vi "Periodic Tasks.vi"(8 "error in":errorcluster) -> ()   [LabVIEW 2014]
doc: "This VI runs in parallel to other tasks. It can contain as many user-defined periodic loops as you need. These can carry out PID or other sorts of timed response."
uses:
  TypeDefs/SRE Enum.ctl
  <vilib>/Rock Robotics/Network Tables/SD Write Number.vi
  Robot Global Data.vi
  Get Ctrl/Get ctrl Secondary axis.vi
  Get Ctrl/Get ctrl Secondary Button.vi
panel:
  in  "Lift to Running":bool
  out "Enum":enum16{"In", "Out", "Done"}(ring)
  in  "Max Change":dbl=0.1
  in  "Stall Speed":dbl=0.05
  out "Angle":dbl
  out "Arm Pot":dbl
  out "Lift Pot":dbl
  out "current (A)":dbl
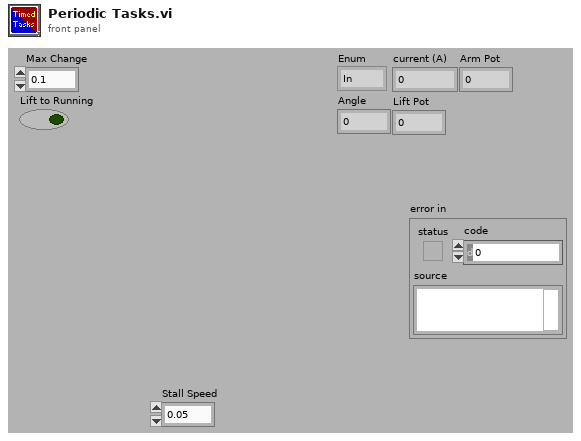
[diagram p1: front panel]
types:
  T1 = enum16{"High", "Middle", "Low", "Really Low", "Stopped"}
  T2 = typedef "SRE Enum.ctl" = enum16{"Start", "Run", "End"}
  T3 = cluster{"proportional gain (Kc)":dbl, "derivative time (Td, min)":dbl}
  T4 = enum16{"manual Control of arm", "manual Control of Elevator", "Output Control"}[]
  T5 = cluster{"Speed":dbl, "Direction":dbl, "Rotation":dbl}
  T6 = enum16{"Auto Stack", "Claw up", "Enable Manuel Elevator", "EM Claw", "Open Claw"}[]
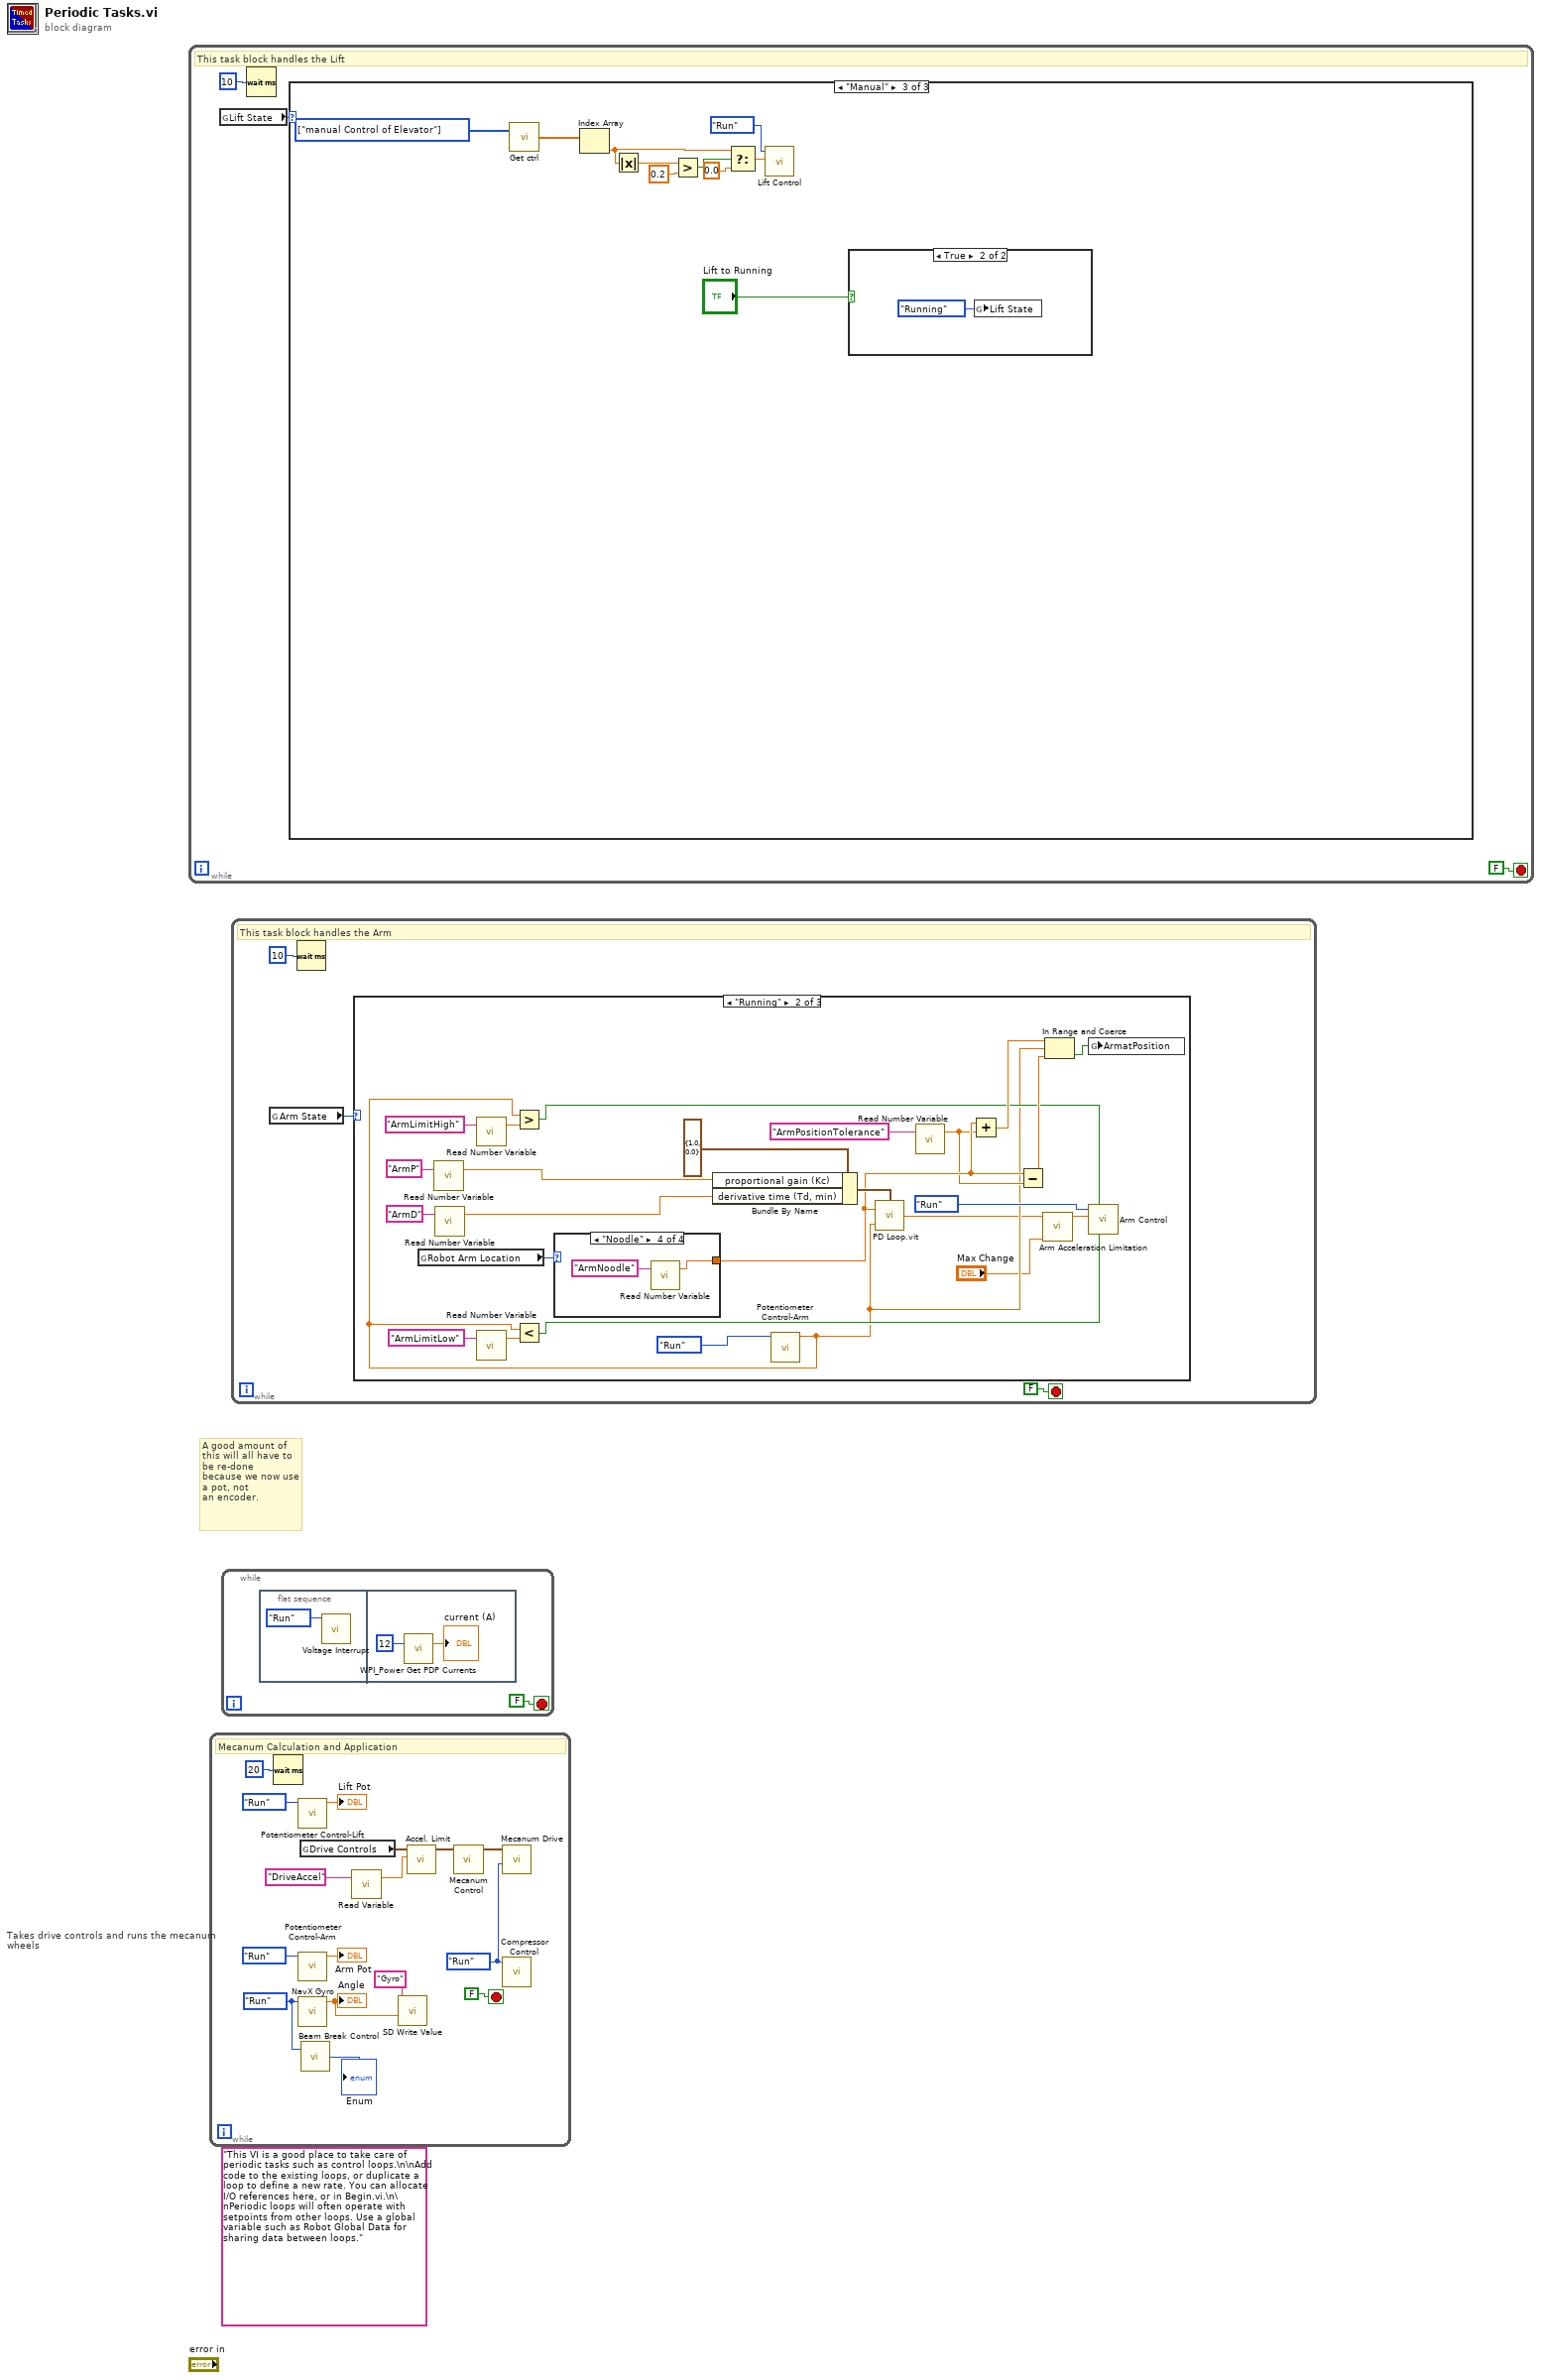
[diagram p0: block diagram]
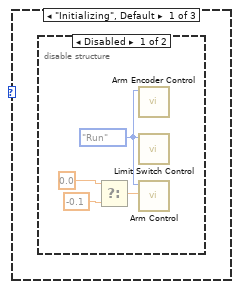
[diagram p2: hidden frame]
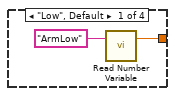
[diagram p4: hidden frame]
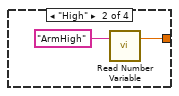
[diagram p5: hidden frame]
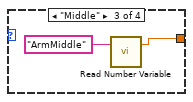
[diagram p6: hidden frame]
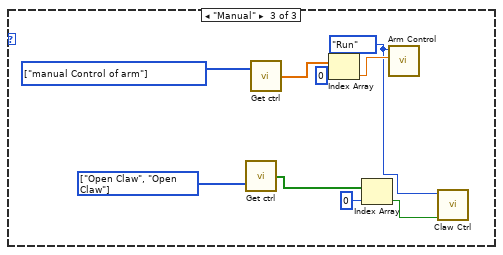
[diagram p7: hidden frame]
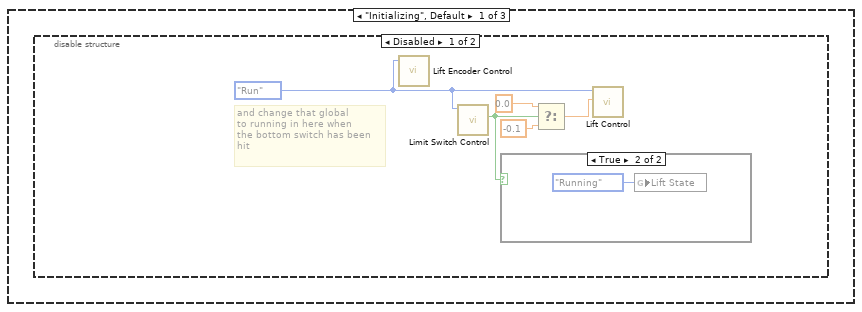
[diagram p8: hidden frame]
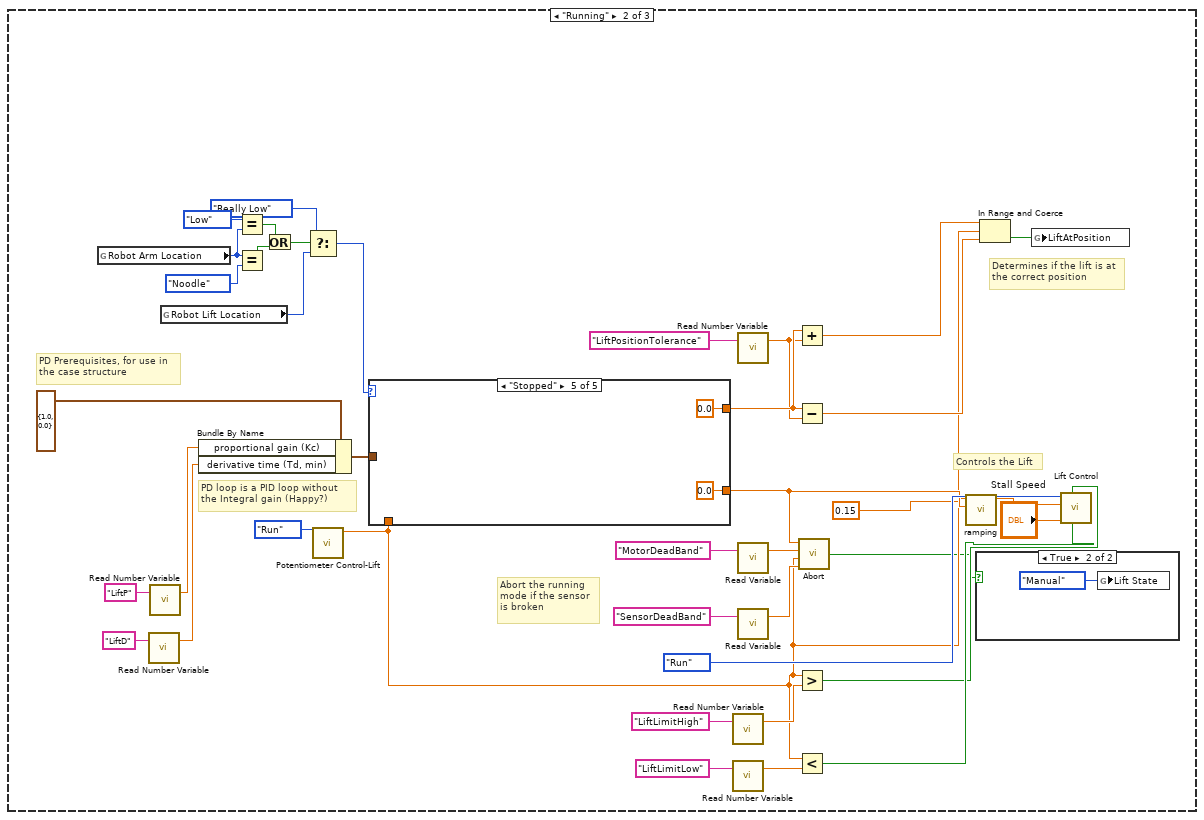
[diagram p11: hidden frame]
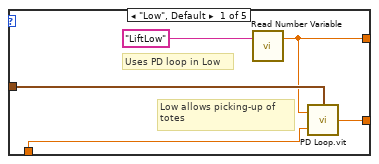
[diagram p13: hidden frame]
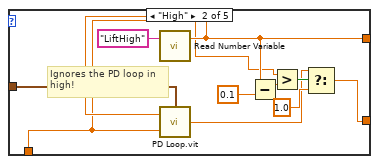
[diagram p14: hidden frame]
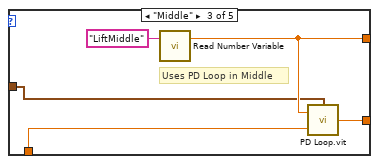
[diagram p15: hidden frame]
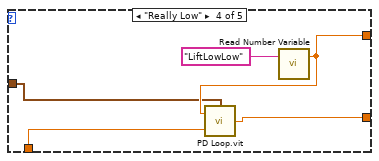
[diagram p16: hidden frame]
diagram:
  (unwired) "This VI is a good place to take care of periodic tasks such as control loops.\n\nAdd code to the existing loops, or duplicate a loop to define a new rate. You can allocate I/O references here, or in Begin.vi.\n\nPeriodic loops will often operate with setpoints from other loops. Use a global variable such as Robot Global Data for sharing data between loops."
  # "A good amount of this will all have to be re-done\nbecause we now use a pot, not\nan encoder."
  n1 = while {
    stop <- FALSE stop-if-true
    # "This task block handles the Lift"
    n2 = global read "Robot Global Data.vi" "Lift State"() -> (w1:enum16{"Initializing", "Running", "Manual"})
    n3 = Wait (ms)(milliseconds to wait=u32 10) -> ()  [unwired: 1 out]
    n4 = case shown="\"Manual\"" w1 {
      frame "Initializing", Default {
        n5 = disable-structure shown="Disabled" {
          frame Disabled {
            w6 = SRE_Enum."Run" ("Enum")
            # "and change that global\nto running in here when\nthe bottom switch has been\nhit"
            n6 = call "Lift Encoder Control.vi"("Enum"=w6) -> ()  [unwired: 6 in, 2 out]
            n7 = call "Limit Switch Control.vi"("Run Mode"=w6) -> ("Lift Bottom"=w4:bool)  [unwired: 7 in, 3 out]
            n8 = case shown="True" w4 {
              frame False {
              }
              frame True {
                n9 = global write "Robot Global Data.vi" "Lift State"(enum16{"Initializing", "Running", "Manual"}."Running" ("Lift State")) -> ()
              }
            }
            n10 = Select(t=0.0, s=w4, f=-0.1) -> (s? t:f=w5:dbl)
            n11 = call "Lift Control.vi"("Motor"=w5, "Enum"=w6) -> ()  [unwired: 9 in, 1 out]
          }
          frame Enabled {
          }
        }
      }
      frame "Running" {
        # "Abort the running\nmode if the sensor\nis broken"
        # "Controls the Lift"
        # "PD loop is a PID loop without\nthe Integral gain (Happy?)"
        # "Determines if the lift is at\nthe correct position"
        # "PD Prerequisites, for use in\nthe case structure"
        n12 = global read "Robot Global Data.vi" "Robot Arm Location"() -> (w20:enum16{"High", "Middle", "Low", "Noodle"})
        n13 = call "Read Number Variable.vi"("Name"="LiftD") -> ("number"=w21:dbl)  [unwired: 1 in, 1 out]
        n14 = call "Read Number Variable.vi"("Name"="LiftP") -> ("number"=w22:dbl)  [unwired: 1 in, 1 out]
        n15 = global read "Robot Global Data.vi" "Robot Lift Location"() -> (w14:T1)
        n16 = Bundle By Name(cluster=T3 {"proportional gain (Kc)"=1.0, "derivative time (Td, min)"=0.0} ("PID gains"), "proportional gain (Kc)"=w22, "derivative time (Td, min)"=w21) -> (w28:T3)
        n17 = Equal?(x=enum16{"High", "Middle", "Low", "Noodle"}."Low", y=w20) -> (x = y?=w16:bool)
        n18 = Equal?(x=w20, y=enum16{"High", "Middle", "Low", "Noodle"}."Noodle") -> (x = y?=w17:bool)
        n19 = Or(x=w16, y=w17) -> (x .or. y?=w15:bool)
        n20 = Select(t=T1."Really Low", s=w15, f=w14) -> (s? t:f=w12:T1)
        n21 = call "Potentiometer Control-Lift.vi"("Enum"=SRE_Enum."Run") -> ("Normalized Value"=w11:dbl)  [unwired: 10 in]
        n22 = case shown="\"Stopped\"" w12 {
          tunnel: [w51 w59 w68 w72 0.0 ("number")] -> w44
          tunnel: w28 -> [w52 w60 w67 w71 _]
          tunnel: [w53 w61 w66 w70 0.0 ("Out Power")] -> w27
          tunnel: w11 -> [w50 w58 w65 w73 _]
          frame "Low", Default {
            # "Low allows picking-up of\ntotes"
            # "Uses PD loop in Low"
            n23 = call "Read Number Variable.vi"("Name"="LiftLow") -> ("number"=w51:dbl)  [unwired: 1 in, 1 out]
            n24 = call "PD Loop.vit"("PD Gains"=w52, "Current"=w50, "Set"=w51) -> ("Out Power"=w53:dbl)
          }
          frame "High" {
            # "Ignores the PD loop in\nhigh!"
            n25 = call "Read Number Variable.vi"("Name"="LiftHigh") -> ("number"=w59:dbl)  [unwired: 1 in, 1 out]
            n26 = call "PD Loop.vit"("PD Gains"=w60, "Current"=w58, "Set"=w59) -> ("Out Power"=w57:dbl)
            n27 = Subtract(x=w59, y=0.1) -> (x-y=w56:dbl)
            n28 = Greater?(x=w58, y=w56) -> (0:w63:bool)
            n29 = Select(t=w57, s=w63, f=1.0) -> (s? t:f=w61:dbl)
          }
          frame "Middle" {
            # "Uses PD Loop in Middle"
            n30 = call "Read Number Variable.vi"("Name"="LiftMiddle") -> ("number"=w68:dbl)  [unwired: 1 in, 1 out]
            n31 = call "PD Loop.vit"("PD Gains"=w67, "Current"=w65, "Set"=w68) -> ("Out Power"=w66:dbl)
          }
          frame "Really Low" {
            n32 = call "Read Number Variable.vi"("Name"="LiftLowLow") -> ("number"=w72:dbl)  [unwired: 1 in, 1 out]
            n33 = call "PD Loop.vit"("PD Gains"=w71, "Current"=w73, "Set"=w72) -> ("Out Power"=w70:dbl)
          }
          frame "Stopped" {
          }
        }
        n34 = call "Read Number Variable.vi"("Name"="LiftLimitHigh") -> ("number"=w46:dbl)  [unwired: 1 in, 1 out]
        n35 = call "Read Number Variable.vi"("Name"="LiftLimitLow") -> ("number"=w45:dbl)  [unwired: 1 in, 1 out]
        n36 = call "Read Number Variable.vi"("Name"="LiftPositionTolerance") -> ("number"=w42:dbl)  [unwired: 1 in, 1 out]
        n37 = call-poly "Read Variable.vi"("Name"="MotorDeadBand") -> ("number"=w38:dbl)  [unwired: 1 in, 1 out]
        n38 = call-poly "Read Variable.vi"("Name"="SensorDeadBand") -> ("number"=w39:dbl)  [unwired: 1 in, 1 out]
        n39 = Add(x=w44, y=w42) -> (x+y=w36:dbl)
        n40 = Subtract(x=w44, y=w42) -> (x-y=w35:dbl)
        n41 = Greater?(x=w11, y=w46) -> (0:w32:bool)
        n42 = Less?(x=w11, y=w45) -> (x < y?=w33:bool)
        n43 = call "Abort.vi"("Sensor Deadband"=w39, "Sensor"=w11, "Motor Deadband"=w38, "Motor"=w27) -> ("Abort"=w10:bool)
        n44 = call "ramping.vi"("Speed"=w27, "Max Change"=0.15) -> ("New Speed"=w26:dbl)  [unwired: 9 in]
        n45 = case shown="True" w10 {
          frame False {
          }
          frame True {
            n46 = global write "Robot Global Data.vi" "Lift State"(enum16{"Initializing", "Running", "Manual"}."Manual" ("Lift State")) -> ()
          }
        }
        n47 = In Range and Coerce(upper limit=w36, x=w11, lower limit=w35) -> (In Range?=w34:bool)  [unwired: 1 out]
        n48 = global write "Robot Global Data.vi" "LiftAtPosition"(w34) -> ()
        n49 = call "Lift Control.vi"("bottom"=w33, "top"=w32, "Stall Speed"="Stall Speed", "Motor"=w26, "Enum"=SRE_Enum."Run") -> ()  [unwired: 6 in, 1 out]
      }
      frame "Manual" {
        w78 = T4 [enum."manual Control of Elevator"] items=["manual Control of arm", "manual Control of Elevator", "Output Control"] ("TypeDef")
        n50 = call-poly "Get ctrl.vi"("TypeDef"=w78) -> ("Array"=w85:dbl[])  [unwired: 2 in]
        n51 = Index Array(array=w85) -> (element=w81:dbl)  [unwired: 1 in]
        n52 = Absolute Value(x=w81) -> (abs(x)=w84:dbl)
        n53 = Greater?(x=w84, y=0.2) -> (0:w82:bool)
        n54 = Select(t=w81, s=w82, f=0.0) -> (s? t:f=w79:dbl)
        n55 = call "Lift Control.vi"("Motor"=w79, "Enum"=SRE_Enum."Run") -> ()  [unwired: 9 in, 1 out]
        n56 = case shown="True" "Lift to Running" {
          frame False {
          }
          frame True {
            n57 = global write "Robot Global Data.vi" "Lift State"(enum16{"Initializing", "Running", "Manual"}."Running" ("Lift State")) -> ()
          }
        }
      }
    }
  }
  n58 = while "Takes drive controls and runs the mecanum wheels" {
    stop <- FALSE stop-if-true
    w89 = SRE_Enum."Run" ("Enum")
    w96 = SRE_Enum."Run" ("Enum")
    # "Mecanum Calculation and Application"
    n59 = Wait (ms)(milliseconds to wait=u32 20) -> ()  [unwired: 1 out]
    n60 = call "Potentiometer Control-Lift.vi"("Enum"=SRE_Enum."Run") -> ("Normalized Value"=→"Lift Pot":dbl)  [unwired: 10 in]
    n61 = call "Potentiometer Control-Arm.vi"("Enum"=SRE_Enum."Run") -> ("Normalized Value"=→"Arm Pot":dbl)  [unwired: 10 in]
    n62 = call "NavX Gyro.vi"("Enum"=w89) -> ("Angle"=w90:dbl)  [unwired: 9 in, 1 out]
    "Angle" <- w90
    n63 = global read "Robot Global Data.vi" "Drive Controls"() -> (w100:T5)
    n64 = call "Beam Break Control.vi"("SRE"=w89) -> ("Enum"=→"Enum":enum16{"In", "Out", "Done"})  [unwired: 2 in]
    n65 = call-poly "Read Variable.vi"("Name"="DriveAccel") -> ("number"=w97:dbl)  [unwired: 1 in, 1 out]
    n66 = call-poly <vilib>:"SD Write Value.vi"("Numeric"=w90, "Name"="Gyro") -> ()  [unwired: 8 in, 2 out]
    n67 = call "Accel. Limit.vi"("Max Change"=w97, "Drive Controls"=w100) -> ("Drive Controls 2"=w99:T5)  [unwired: 9 in]
    n68 = call "Mecanum Control.vi"("Drive Controls"=w99) -> ("Wheel m's"=w101:cluster{dbl, dbl, dbl, dbl})  [unwired: 10 in]
    n69 = call "Mecanum Drive.vi"("Enum"=w96, "Motor Power"=w101) -> ()  [unwired: 10 in]
    n70 = call "Compressor Control.vi"("Mode"=w96) -> ()  [unwired: 11 in]
  }
  n71 = while {
    stop <- FALSE stop-if-true
    n72 = flat-sequence {
      frame #0 {
        n73 = call "Voltage Interrupt.vi"("Enum"=SRE_Enum."Run") -> ()  [unwired: 11 in]
      }
      frame #1 {
        n74 = call <vilib>:"WPI_Power Get PDP Currents.vi"("PDP Channel"=12) -> ("current (A)"=→"current (A)":dbl)  [unwired: 12 in, 2 out]
      }
    }
  }
  n75 = while {
    stop <- FALSE stop-if-true
    # "This task block handles the Arm"
    n76 = global read "Robot Global Data.vi" "Arm State"() -> (w108:enum16{"Initializing", "Running", "Manual"})
    n77 = Wait (ms)(milliseconds to wait=u32 10) -> ()  [unwired: 1 out]
    n78 = case shown="\"Running\"" w108 {
      frame "Initializing", Default {
        n79 = disable-structure shown="Disabled" {
          frame Disabled {
            w111 = SRE_Enum."Run" ("Enum")
            n80 = Select(t=0.0, f=-0.1) -> (s? t:f=w112:dbl)  [unwired: 1 in]
            n81 = call "Arm Encoder Control.vi"("Enum"=w111) -> ()  [unwired: 9 in, 2 out]
            n82 = call "Limit Switch Control.vi"("Run Mode"=w111) -> ()  [unwired: 7 in, 4 out]
            n83 = call "Arm Control.vi"("Motor"=w112, "Enum"=w111) -> ()  [unwired: 10 in]
          }
          frame Enabled {
          }
        }
      }
      frame "Running" {
        n84 = global read "Robot Global Data.vi" "Robot Arm Location"() -> (w130:enum16{"High", "Middle", "Low", "Noodle"})
        n85 = call "Read Number Variable.vi"("Name"="ArmP") -> ("number"=w119:dbl)  [unwired: 1 in, 1 out]
        n86 = call "Read Number Variable.vi"("Name"="ArmD") -> ("number"=w118:dbl)  [unwired: 1 in, 1 out]
        n87 = call "Read Number Variable.vi"("Name"="ArmLimitHigh") -> ("number"=w134:dbl)  [unwired: 1 in, 1 out]
        n88 = call "Read Number Variable.vi"("Name"="ArmLimitLow") -> ("number"=w133:dbl)  [unwired: 1 in, 1 out]
        n89 = case shown="\"Noodle\"" w130 {
          tunnel: [w140 w142 w144 w146] -> w125
          frame "Low", Default {
            n90 = call "Read Number Variable.vi"("Name"="ArmLow") -> ("number"=w140:dbl)  [unwired: 1 in, 1 out]
          }
          frame "High" {
            n91 = call "Read Number Variable.vi"("Name"="ArmHigh") -> ("number"=w142:dbl)  [unwired: 1 in, 1 out]
          }
          frame "Middle" {
            n92 = call "Read Number Variable.vi"("Name"="ArmMiddle") -> ("number"=w144:dbl)  [unwired: 1 in, 1 out]
          }
          frame "Noodle" {
            n93 = call "Read Number Variable.vi"("Name"="ArmNoodle") -> ("number"=w146:dbl)  [unwired: 1 in, 1 out]
          }
        }
        n94 = Bundle By Name(cluster=T3 {"proportional gain (Kc)"=1.0, "derivative time (Td, min)"=0.0} ("PID gains"), "proportional gain (Kc)"=w119, "derivative time (Td, min)"=w118) -> (w131:T3)
        n95 = call "Potentiometer Control-Arm.vi"("Enum"=SRE_Enum."Run" ("Run Mode")) -> ("Normalized Value"=w120:dbl)  [unwired: 10 in]
        n96 = Greater?(x=w120, y=w134) -> (0:w121:bool)
        n97 = Less?(x=w120, y=w133) -> (x < y?=w122:bool)
        n98 = call "PD Loop.vit"("PD Gains"=w131, "Current"=w120, "Set"=w125) -> ("Out Power"=w115:dbl)
        n99 = call "Read Number Variable.vi"("Name"="ArmPositionTolerance") -> ("number"=w124:dbl)  [unwired: 1 in, 1 out]
        n100 = Add(x=w125, y=w124) -> (x+y=w127:dbl)
        n101 = Subtract(x=w125, y=w124) -> (x-y=w123:dbl)
        n102 = call "Arm Acceleration Limitation.vi"("Max Change"="Max Change", "Input"=w115) -> ("New Speed"=w116:dbl)  [unwired: 9 in]
        n103 = In Range and Coerce(upper limit=w127, x=w120, lower limit=w123) -> (In Range?=w126:bool)  [unwired: 1 out]
        n104 = global write "Robot Global Data.vi" "ArmatPosition"(w126) -> ()
        n105 = call "Arm Control.vi"("bottom"=w122, "top"=w121, "Motor"=w116, "Enum"=SRE_Enum."Run") -> ()  [unwired: 8 in]
      }
      frame "Manual" {
        w152 = T6 [enum."Open Claw", enum."Open Claw"] items=["Auto Stack", "Claw up", "Enable Manuel Elevator", "EM Claw", "Open Claw"] ("Controls")
        w156 = T4 [enum."manual Control of arm"] items=["manual Control of arm", "manual Control of Elevator", "Output Control"] ("TypeDef")
        w148 = SRE_Enum."Run" ("Enum")
        n106 = call-poly "Get ctrl.vi"("Controls"=w152) -> ("Array"=w151:bool[])  [unwired: 2 in]
        n107 = call-poly "Get ctrl.vi"("TypeDef"=w156) -> ("Array"=w154:dbl[])  [unwired: 2 in]
        n108 = Index Array(array=w154, index=0) -> (element=w153:dbl)
        n109 = Index Array(array=w151, index=0) -> (element=w149:bool)
        n110 = call "Arm Control.vi"("Motor"=w153, "Enum"=w148) -> ()  [unwired: 10 in]
        n111 = call "Claw Ctrl.vi"("Open/Close"=w149, "Enum"=w148) -> ()  [unwired: 10 in]
      }
    }
  }
